vi "start.vi"(8 "error in (no error)":errorcluster, 10 "enable_event":bool, 11 "queue_size":i32=10) -> (0 "error out":errorcluster, 3 "references":T1)   [LabVIEW 2015, in "repub-dvr_nre.lvlib"]
doc: "This VI can be used to asynchronously start (and stop) the main of its module/library. This is neat, but can be confusing, alternatively, you could run the module on a higher level main. If false, it'll start the module and block until the references are created. If true, it will stop the module and wait until the main has stopped running."
uses:
  repub-dvr_nre.lvlib
  private/_controls/input_command.ctl
  _controls/configuration.ctl
  private/_controls/input.ctl
  private/_controls/output.ctl
  private/_controls/data.ctl
  _controls/references.ctl
  _controls/change.ctl
  lv-recipe-machine/public/_controls/automatic_state.ctl
  lv-recipe-machine/lv-recipe-machine.lvlib
  lv-recipe-machine/public/_controls/manual_state.ctl
  lv-recipe-machine/public/_controls/mode.ctl
  lv-recipe-machine/private/_controls/recipe_data.ctl
  <userlib>/antonio-alexander/lv-waitgroup/public/_controls/api_waitgroup.ctl
  <userlib>/antonio-alexander/lv-waitgroup/lv-waitgroup.lvlib
  lv-recipe-machine/public/_controls/transition.ctl
  _controls/status.ctl
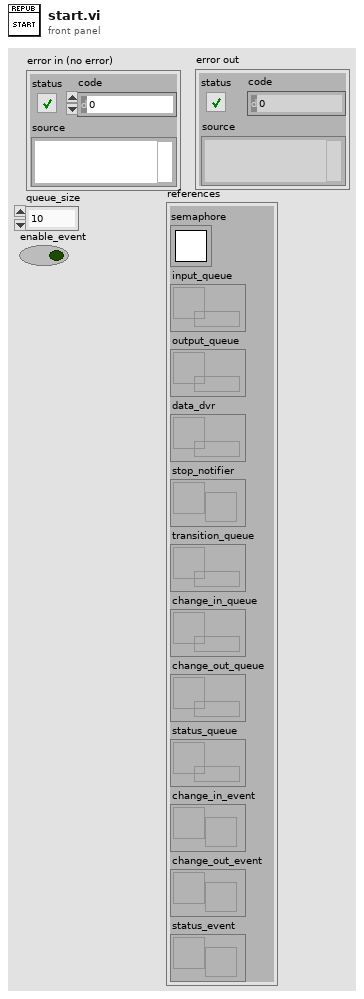
[diagram p1: front panel]
types:
  T1 = typedef "repub-dvr_nre.lvlib/references.ctl" = cluster{"semaphore":T2, "input_queue":refnum<queue>, "output_queue":refnum<queue>, "data_dvr":refnum<data-value>, "stop_notifier":refnum<notifier>, "transition_queue":refnum<queue>, "change_in_queue":refnum<queue>, "change_out_queue":refnum<queue>, "status_queue":refnum<queue>, "change_in_event":refnum<user-event>, "change_out_event":refnum<user-event>, "status_event":refnum<user-event>}
  T2 = typedef "Semaphore RefNum" = refnum<k1>
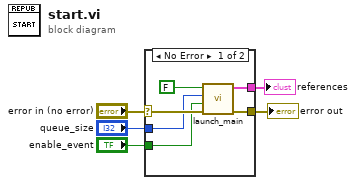
[diagram p0: block diagram]
diagram:
  n1 = case shown="No Error" "error in (no error)" {
    selector: "error in (no error)" -> [w9 w12]
    tunnel: [w11 w12] -> w4
    tunnel: [w8 _] -> w3
    tunnel: "queue_size" -> [w7 _]
    tunnel: "enable_event" -> [w6 _]
    frame No Error {
      n2 = call "launch_main.vi"("error in (no error)"=w9, "enable_event"=w6, "queue_size"=w7, "run_f_stop_t"=FALSE ("Run(F)/Abort(T)")) -> ("error out"=w11:errorcluster, "references"=w8:T1)  [unwired: 6 in]
    }
    frame Error {
    }
  }
  "error out" <- w4
  "references" <- w3
